vi "PH_PowerUnit_BaseClass.SM scr.vi"(0 "VI in":refnum<vi>, 1 "Current SM State (condition)":T1, 2 "Wanted SM State":T1, 3 "Further change condition":bool, 4 "PU in use is condition? (true)":bool=TRUE, 5 "error in (no error)":errorcluster) -> (14 "VI out":refnum<vi>, 19 "error out":errorcluster)   [LabVIEW 2014, in "PH_PowerUnit_BaseClass.lvlib"]
doc: "This VI requests a state change of the state machine if conditions are right to change."
uses:
  PH_PowerUnit_BaseClass.lvlib
  PH_PowerUnit_BaseClass.SM States.ctl
  CS_Core/BaseSM/BaseSM.lvlib
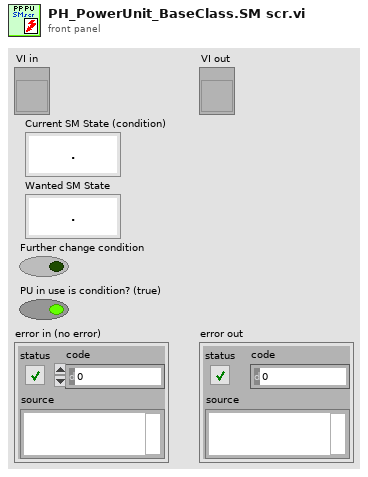
[diagram p1: front panel]
types:
  T1 = typedef "PH_PowerUnit_BaseClass.lvlib/PH_PowerUnit_BaseClass.SM States.ctl" = enum16{".", "Stand by", "Switch PU on", "Configure", "Set Default Voltage", "Set STANDBY", "Set READY", "Wait for Shot Cmd", "Open Dump Rods", "Open Ross Relais", "Close Ross Relais", "Switch PSU on", "Switch PSU off", "Charge", "Switch GD Channel on", "Close Dump Rods", "Rods-TO", "RR-TO", "PSU-TO", "Trigger-TO"}
  T2 = typedef "PH_PowerUnit_BaseClass.lvlib/PH_PowerUnit_BaseClass.i attribute.ctl" = cluster{"Constructor finished":bool, "PU":cluster{"In use":bool, "Service ID in use":i32, "GUI Ref":refnum<vi>}, "Enabling":cluster{"State":T3, "GUI Ref":refnum<vi>}, "Timing":cluster{"Last Shot":dbl, "Time between Shots [Sec]":dbl, "Waiting Time over?":bool, "Service ID Waiting Time":i32, "GUI Ref":refnum<vi>, "Instance":cluster{"Status":T4, "linked?":bool, "GUI Ref":refnum<vi>}}, "Sequencer":cluster{"SM State":string, "GUI Ref":refnum<vi>, "linked":bool}, "Subscribed Trendmssgs":cluster{"Tagname":string, "Status":T4, "linked?":bool, "Shot Condition":T4, "GUI Ref":refnum<vi>}[], "PP PU":T5, "Default Voltage (V)":dbl, "GUI Refs":T6, "PSDB data":cluster{"Shot Voltage [V]":dbl, "State TO SM":T1, "Write 2 early":bool}, "State TO SM":T1}
  T3 = typedef "PH_SystemInformation.lvlib/PH_SystemInformationEnabling State.ctl" = i32
  T4 = typedef "PH_StatusHandler.lvlib/PH_StatusHandler.Status.ctl" = i16
  T5 = typedef "PH_PP_Common.lvlib/PH_PP_Common.PUs.ctl" = enum16{"no Info", "PA-19mm-1", "PA-19mm-2", "PA-45mm-PILC", "PA-45mm-MAIN", "MA-PU-1", "MA-PU-2", "MA-PU-3", "MA-PU-4", "MA-PU-5", "MA-PU-6", "MA-FR", "MA-PILC", "PA-45mm-DP"}
  T6 = typedef "PH_PowerUnit_BaseClass.lvlib/PH_PowerUnit_BaseClass.GUI Refs.ctl" = cluster{"Delete Inst":refnum<vi>, "State TO SM":refnum<vi>, "State SM":refnum<vi>, "Fire":refnum<vi>}
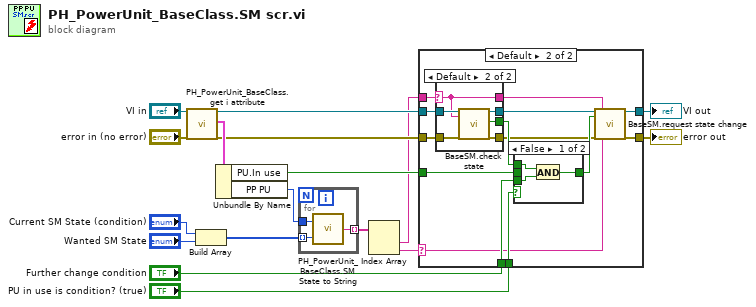
[diagram p0: block diagram]
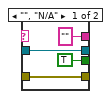
[diagram p3: hidden frame]
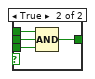
[diagram p4: hidden frame]
diagram:
  n1 = call "PH_PowerUnit_BaseClass.get i attribute.vi"("i ref in"="VI in", "error in (no error)"="error in (no error)") -> ("i ref out"=w7:refnum<vi>, "i attribute"=w10:T2, "error out"=w9:errorcluster)  [unwired: 15 in]
  n2 = Build Array("Current SM State (condition)", "Wanted SM State") -> (w15:T1[])
  n3 = Unbundle By Name(w10) -> ("PU.In use"=w13:bool, "PP PU"=w11:T5)
  n4 = for {
    tunnel: w11 -> [w20]
    tunnel: w15 -> [w19] mode=indexing
    tunnel: [w18] -> w17 mode=indexing
    n5 = call "PH_PowerUnit_BaseClass.SM State to String.vi"("SM State"=w19, "PU"=w20) -> ("SM State String"=w18:string)
  }
  n6 = Index Array(array=w17) -> (element #1=w2:string, element #2=w1:string)  [unwired: 2 in]
  n7 = case shown="Default" w1 {
    selector: w1 -> [_ w23]
    tunnel: "PU in use is condition? (true)" -> [_ w36]
    tunnel: w13 -> [_ w35]
    tunnel: w9 -> [w21 w34]
    tunnel: w7 -> [w22 w33]
    tunnel: "Further change condition" -> [_ w31]
    tunnel: [w21 w27] -> w4
    tunnel: [w22 w26] -> w3
    tunnel: w2 -> [_ w25]
    frame "", "N/A" {
    }
    frame Default {
      n8 = case shown="Default" w25 {
        selector: w25 -> [_ w41]
        tunnel: w34 -> [w38 w46]
        tunnel: w33 -> [w39 w45]
        tunnel: [TRUE ("OK") w44] -> w30
        tunnel: [w38 w43] -> w29
        tunnel: [w39 w42] -> w28
        tunnel: ["" w41] -> w24
        frame "", "N/A" {
        }
        frame Default {
          n9 = call "BaseSM.check state.vi"("i ref in"=w45, "requestedState"=w41, "error in (no error)"=w46) -> ("i ref out"=w42:refnum<vi>, "OK"=w44:bool, "error out"=w43:errorcluster)  [unwired: 11 in, 3 out]
        }
      }
      n10 = case shown="False" w36 {
        tunnel: w30 -> [w49 w53]
        tunnel: w31 -> [w48 w50]
        tunnel: [w47 w52] -> w32
        tunnel: w35 -> [_ w51]
        frame False {
          n11 = And(x=w49, y=w48) -> (x .and. y?=w47:bool)
        }
        frame True {
          n12 = Compound Arithmetic op=AND(w53, w51, w50) -> (w52:bool)
        }
      }
      n13 = call "BaseSM.request state change.vi"("i ref in"=w28, "change"=w32, "error in (no error)"=w29, "allowed current state"=w24, "requested state"=w23) -> ("i ref out"=w26:refnum<vi>, "error out"=w27:errorcluster)  [unwired: 11 in, 2 out]
    }
  }
  "error out" <- w4
  "VI out" <- w3
